vi "2LOOPs-DAQ.vi"() -> ()   [LabVIEW 2020]
uses:
  <vilib>/ptbypt/NI_PtbyPt.lvlib
panel:
  out "Chart":dbl(graph)
  in  "PauseDAQ":bool
  in  "StartDAQ":bool
  out "ErrO":errorcluster
  in  "ErrI":errorcluster
  in  "Exit":bool
  # "Messages will be sent\nto DAQ Loop to contol\nthe DAQ Start / Pause."
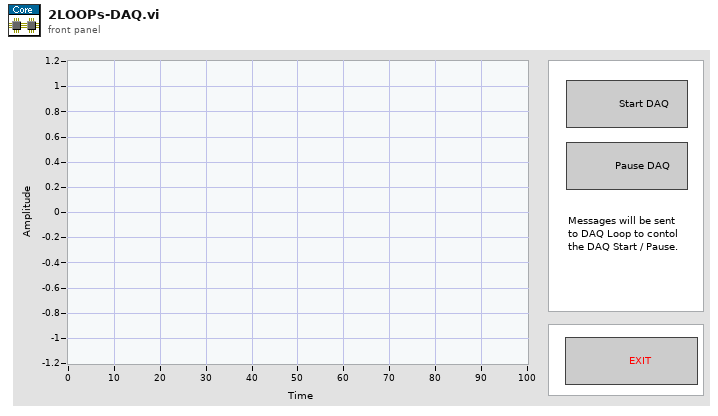
[diagram p1: front panel]
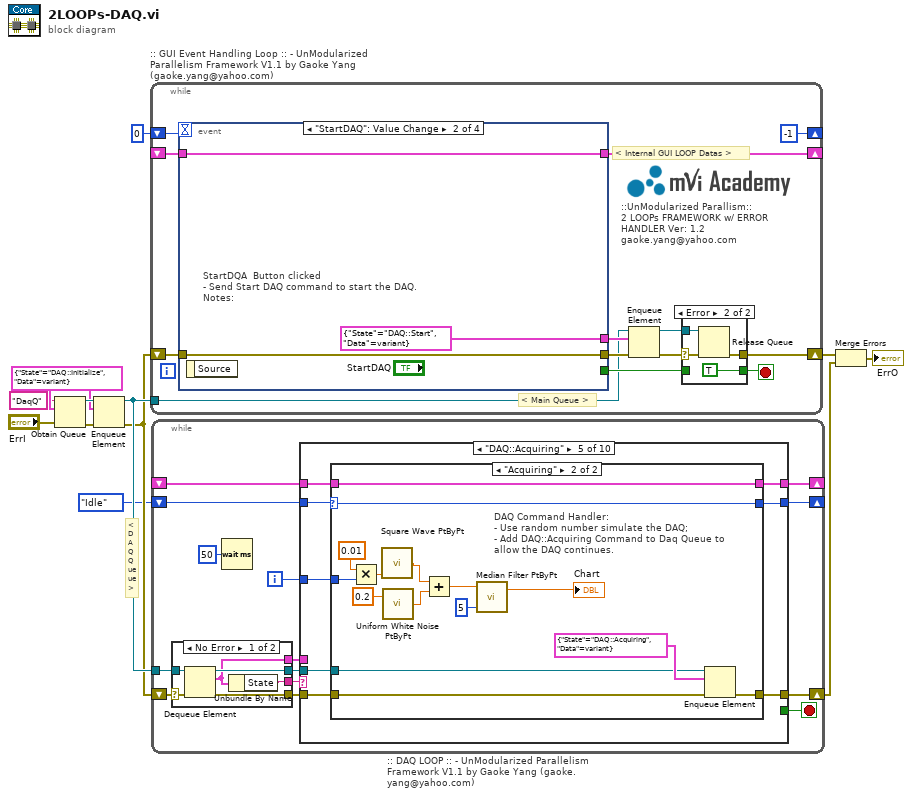
[diagram p0: block diagram]
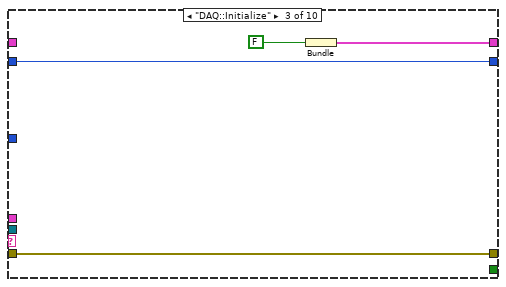
[diagram p4: hidden frame]
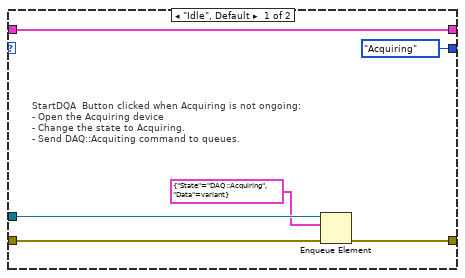
[diagram p6: hidden frame]
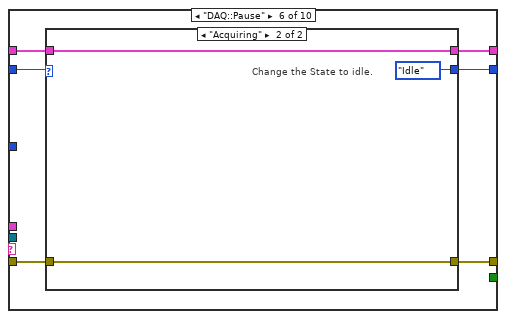
[diagram p8: hidden frame]
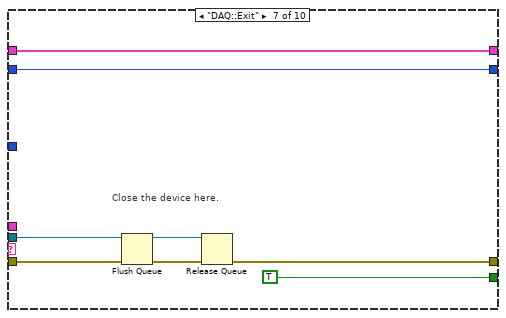
[diagram p10: hidden frame]
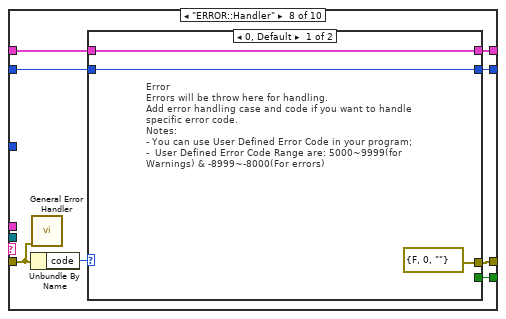
[diagram p11: hidden frame]
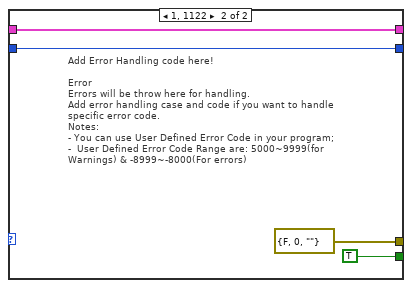
[diagram p12: hidden frame]
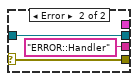
[diagram p15: hidden frame]
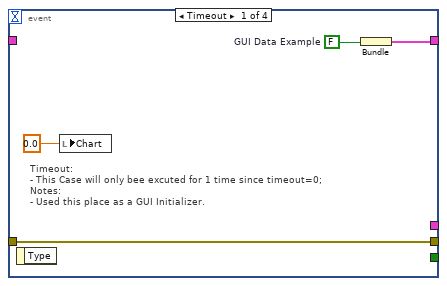
[diagram p17: hidden frame]
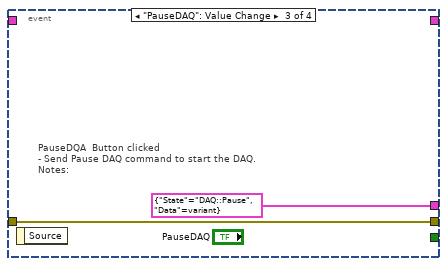
[diagram p18: hidden frame]
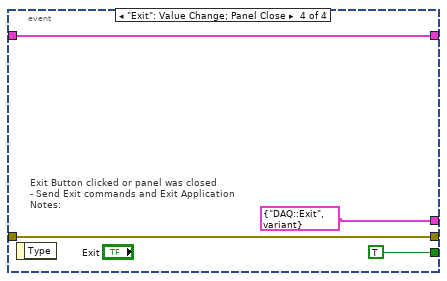
[diagram p19: hidden frame]
diagram:
  w8 = cluster{"State":string, "Data":variant} {"State"="DAQ::Initialize", "Data"=variant} ("MainQueue")
  # "< DAQ Queue >"
  n1 = Obtain Queue(name (unnamed)="DaqQ", element data type=w8, error in (no error)="ErrI") -> (queue out=w10:refnum<queue>, error out=w9:errorcluster)  [unwired: 2 in, 1 out]
  n2 = Enqueue Element(queue=w10, element=w8, error in (no error)=w9) -> (queue out=w6:refnum<queue>, error out=w5:errorcluster)  [unwired: 2 out]
  n3 = while ":: GUI Event Handling Loop :: - UnModularized Parallelism Framework V1.1 by Gaoke Yang (gaoke.yang@yahoo.com)" {
    tunnel: w6 -> [w15]
    shift-right: [w24] -> w12
    shift-left: w5 -> [w25]
    shift-right: [-1] -> _
    shift-left: 0 -> [w22]
    shift-right: [w21] -> _
    shift-left: _ -> [w20]
    stop <- w18 stop-if-true
    # "::UnModularized Parallism::\n2 LOOPs FRAMEWORK w/ ERROR HANDLER Ver: 1.2\ngaoke.yang@yahoo.com"
    # "< Internal GUI LOOP Datas >"
    # "< Main Queue >"
    n4 = event shown="[1] \"StartDAQ\": Value Change" {
      selector: _ -> [_ _ _ _]
      dyn-events: _ -> [_ _ _ _]
      timeout: w22 -> [_ _ _ _]
      tunnel: [_ _ _ TRUE ("Exit")] -> w19
      tunnel: w25 -> [w35 w38 w40 w41]
      tunnel: [w35 w38 w40 w41] -> w17
      tunnel: [_ cluster{"State":string, "Data":variant} {"State"="DAQ::Start", "Data"=variant} ("MainQueue") cluster{"State":string, "Data":variant} {"State"="DAQ::Pause", "Data"=variant} ("MainQueue") cluster{"State":string, "Data":variant} {"State"="DAQ::Exit", "Data"=variant} ("Packet")] -> w16
      tunnel: [w33 w37 _ w44] -> w21
      tunnel: w20 -> [_ w37 _ w44]
      event Timeout {
        w34 = FALSE  # GUI Data Example
        # "Timeout:\n- This Case will only bee excuted for 1 time since timeout=0;\nNotes:\n- Used this place as a GUI Initializer."
        n5 = event-data() -> ()  [unwired: 2 out]
        n6 = local write "Chart"(0.0 ("Chart")) -> ()
        n7 = Bundle("GUI Data Example"=w34) -> (w33:cluster{"GUI Data Example":bool})  [unwired: 1 in]
      }
      event "StartDAQ": Value Change {
        # "StartDQA  Button clicked\n- Send Start DAQ command to start the DAQ.\nNotes:"
        n8 = event-data() -> ()  [unwired: 2 out]
      }
      event "PauseDAQ": Value Change {
        # "PauseDQA  Button clicked\n- Send Pause DAQ command to start the DAQ.\nNotes:"
        n9 = event-data() -> ()  [unwired: 2 out]
      }
      event "Exit": Value Change; Panel Close {
        # "Exit Button clicked or panel was closed\n- Send Exit commands and Exit Application\nNotes:"
        n10 = event-data() -> ()  [unwired: 2 out]
      }
    }
    n11 = Enqueue Element(queue=w15, element=w16, error in (no error)=w17) -> (queue out=w13:refnum<queue>, error out=w14:errorcluster)  [unwired: 2 out]
    n12 = case shown="Error" w14 {
      selector: w14 -> [w27 w30]
      tunnel: [w27 w28] -> w24
      tunnel: w19 -> [w26 _]
      tunnel: [w26 TRUE ("Exit")] -> w18
      tunnel: w13 -> [_ w29]
      frame No Error {
      }
      frame Error {
        n13 = Release Queue(queue=w29, error in (no error)=w30) -> (error out=w28:errorcluster)  [unwired: 1 in, 2 out]
      }
    }
  }
  n14 = while ":: DAQ LOOP :: - UnModularized Parallelism Framework V1.1 by Gaoke Yang (gaoke.yang@yahoo.com)" {
    tunnel: w6 -> [w58]
    shift-right: [w52] -> w4
    shift-left: w5 -> [w57]
    shift-right: [w49] -> _
    shift-left: _ -> [w50]
    shift-right: [w46] -> _
    shift-left: enum16{"Idle", "Acquiring"}."Idle" -> [w47]
    i -> [w45]
    stop <- w51 stop-if-true
    n15 = case shown="No Error" w57 {
      selector: w57 -> [w152 w160]
      tunnel: w58 -> [w157 w158]
      tunnel: [w156 w160] -> w56
      tunnel: [w155 w158] -> w54
      tunnel: [w154 "ERROR::Handler" ("State")] -> w55
      tunnel: [w153 _] -> w53
      frame No Error {
        n16 = Dequeue Element(queue=w157, error in (no error)=w152) -> (queue out=w155:refnum<queue>, element=w153:cluster{"State":string, "Data":variant}, error out=w156:errorcluster)  [unwired: 2 out]
        n17 = Unbundle By Name(w153) -> ("State"=w154:string)
      }
      frame Error {
      }
    }
    n18 = Wait (ms)(milliseconds to wait=u32 50) -> ()  [unwired: 1 out]
    n19 = case shown="\"DAQ::Acquiring\"" w55 {
      tunnel: w56 -> [w60 w64 w66 w74 w91 w112 w129 w134 w148 w151]
      tunnel: [w60 w64 w66 w75 w92 w111 w126 w136 w148 w151] -> w52
      tunnel: [_ _ _ _ _ _ TRUE w135 _ _] -> w51
      tunnel: w54 -> [_ _ _ w73 w90 _ w128 _ _ _]
      tunnel: [w61 w63 w67 w72 w88 w114 w124 w137 w147 w150] -> w49
      tunnel: w50 -> [w61 w63 _ w71 w89 w115 w124 w138 w147 w150]
      tunnel: w53 -> [_ _ _ _ _ _ _ _ _ _]
      tunnel: w47 -> [w59 w62 w65 w70 w87 w113 w123 w132 w146 w149]
      tunnel: [w59 w62 w65 w69 w86 w116 w123 w131 w146 w149] -> w46
      tunnel: w45 -> [_ _ _ _ w85 _ _ _ _ _]
      frame "IDLE", Default {
      }
      frame "-------- DAQ ---------" {
      }
      frame "DAQ::Initialize" {
        n20 = Bundle(FALSE) -> (w67:cluster{bool})  [unwired: 1 in]
      }
      frame "DAQ::Start" {
        n21 = case shown="\"Acquiring\"" w70 {
          selector: w70 -> [_ w82]
          tunnel: [w81 w83] -> w75
          tunnel: w74 -> [w80 w83]
          tunnel: w73 -> [w79 _]
          tunnel: [w77 w84] -> w72
          tunnel: w71 -> [w77 w84]
          tunnel: [enum16{"Idle", "Acquiring"}."Acquiring" w82] -> w69
          frame "Idle", Default {
            # "StartDQA  Button clicked when Acquiring is not ongoing:\n- Open the Acquiring device\n- Change the state to Acquiring.\n- Send DAQ::Acquiting command to queues."
            n22 = Enqueue Element(queue=w79, element=cluster{"State":string, "Data":variant} {"State"="DAQ::Acquiring", "Data"=variant} ("DaqQueue"), error in (no error)=w80) -> (error out=w81:errorcluster)  [unwired: 3 out]
          }
          frame "Acquiring" {
            # "The system is already acquiring. \nIgnore the \"Start\" message."
          }
        }
      }
      frame "DAQ::Acquiring" {
        n23 = case shown="\"Acquiring\"" w87 {
          selector: w87 -> [w94 w105]
          tunnel: [w93 w110] -> w92
          tunnel: w91 -> [w93 w109]
          tunnel: w90 -> [_ w107]
          tunnel: w89 -> [w95 w106]
          tunnel: [w95 w106] -> w88
          tunnel: [w94 w105] -> w86
          tunnel: w85 -> [_ w101]
          frame "Idle", Default {
            # "Ignore \"Acquire\" command when the acquisition is idle."
          }
          frame "Acquiring" {
            # "DAQ Command Handler: \n- Use random number simulate the DAQ;\n- Add DAQ::Acquiring Command to Daq Queue to allow the DAQ continues."
            n24 = Multiply(x=0.01 ("amplitude"), y=w101) -> (x*y=w99:dbl)
            n25 = call <vilib>:"Square Wave PtByPt.vi"("time"=w99) -> ("square wave"=w98:dbl)  [unwired: 4 in]
            n26 = call <vilib>:"Uniform White Noise PtByPt.vi"("amplitude"=0.2) -> ("uniform white noise"=w102:dbl)  [unwired: 2 in]
            n27 = Add(x=w98, y=w102) -> (x+y=w97:dbl)
            n28 = call <vilib>:"Median Filter PtByPt.vi"("rank"=5, "x"=w97) -> ("Filtered x"=→"Chart":dbl)  [unwired: 2 in, 1 out]
            n29 = Enqueue Element(queue=w107, element=cluster{"State":string, "Data":variant} {"State"="DAQ::Acquiring", "Data"=variant} ("DaqQueue"), error in (no error)=w109) -> (error out=w110:errorcluster)  [unwired: 3 out]
          }
        }
      }
      frame "DAQ::Pause" {
        n30 = case shown="\"Acquiring\"" w113 {
          selector: w113 -> [w118 _]
          tunnel: [w118 enum16{"Idle", "Acquiring"}."Idle"] -> w116
          tunnel: w115 -> [w119 w121]
          tunnel: [w119 w121] -> w114
          tunnel: w112 -> [w117 w120]
          tunnel: [w117 w120] -> w111
          frame "Idle", Default {
            # "Already idle, ignore Pause command."
          }
          frame "Acquiring" {
            # "Change the State to idle."
          }
        }
      }
      frame "DAQ::Exit" {
        # "Close the device here."
        n31 = Flush Queue(queue=w128, error in (no error)=w129) -> (queue out=w125:refnum<queue>, error out=w127:errorcluster)  [unwired: 1 out]
        n32 = Release Queue(queue=w125, error in (no error)=w127) -> (error out=w126:errorcluster)  [unwired: 1 in, 2 out]
      }
      frame "ERROR::Handler" {
        n33 = Unbundle By Name(w134) -> ("code"=w133:i32)
        n34 = call <vilib>:"General Error Handler.vi"("error in (no error)"=w134) -> ()  [unwired: 10 in, 5 out]
        n35 = case shown="0, Default" w133 {
          tunnel: [w141 w145] -> w137
          tunnel: w138 -> [w141 w145]
          tunnel: [errorcluster {"status"=FALSE, "code"=0, "source"=""} ("error out") errorcluster {"status"=FALSE, "code"=0, "source"=""} ("error out")] -> w136
          tunnel: [_ TRUE] -> w135
          tunnel: w132 -> [w139 w142]
          tunnel: [w139 w142] -> w131
          frame 0, Default {
            # "Error\nErrors will be throw here for handling.\nAdd error handling case and code if you want to handle specific error code.\nNotes:\n- You can use User Defined Error Code in your program;\n-  User Defined Error Code Range are: 5000~9999(for Warnings) & -8999~-8000(For errors)"
          }
          frame 1, 1122 {
            # "Add Error Handling code here!\n\nError\nErrors will be throw here for handling.\nAdd error handling case and code if you want to handle specific error code.\nNotes:\n- You can use User Defined Error Code in your program;\n-  User Defined Error Code Range are: 5000~9999(for Warnings) & -8999~-8000(For errors)"
          }
        }
      }
      frame "----- User Case ------" {
      }
      frame "Reserved" {
      }
    }
  }
  n36 = Merge Errors(w12, w4) -> (→"ErrO":errorcluster)
